vi "Handler - Set APU&ECU Cntrls.vi"(8 "error in (no error)":errorcluster, 10 "APU & ECU Controls":T1, 11 "Message Handler Loop Data in":T2) -> (0 "error out":errorcluster)   [LabVIEW 2018]
uses:
  Private Controls/Message Handler Loop Data.ctl
  Modules/Testing UI 1/Private Controls/APU & ECU Controls.ctl
  Modules/Testing UI 1/Testing UI 1.lvlib
  FPGA/FPGA VI Reference.ctl
panel:
  # "GTCP331-200ER Control Panel Discrete Input Panel"
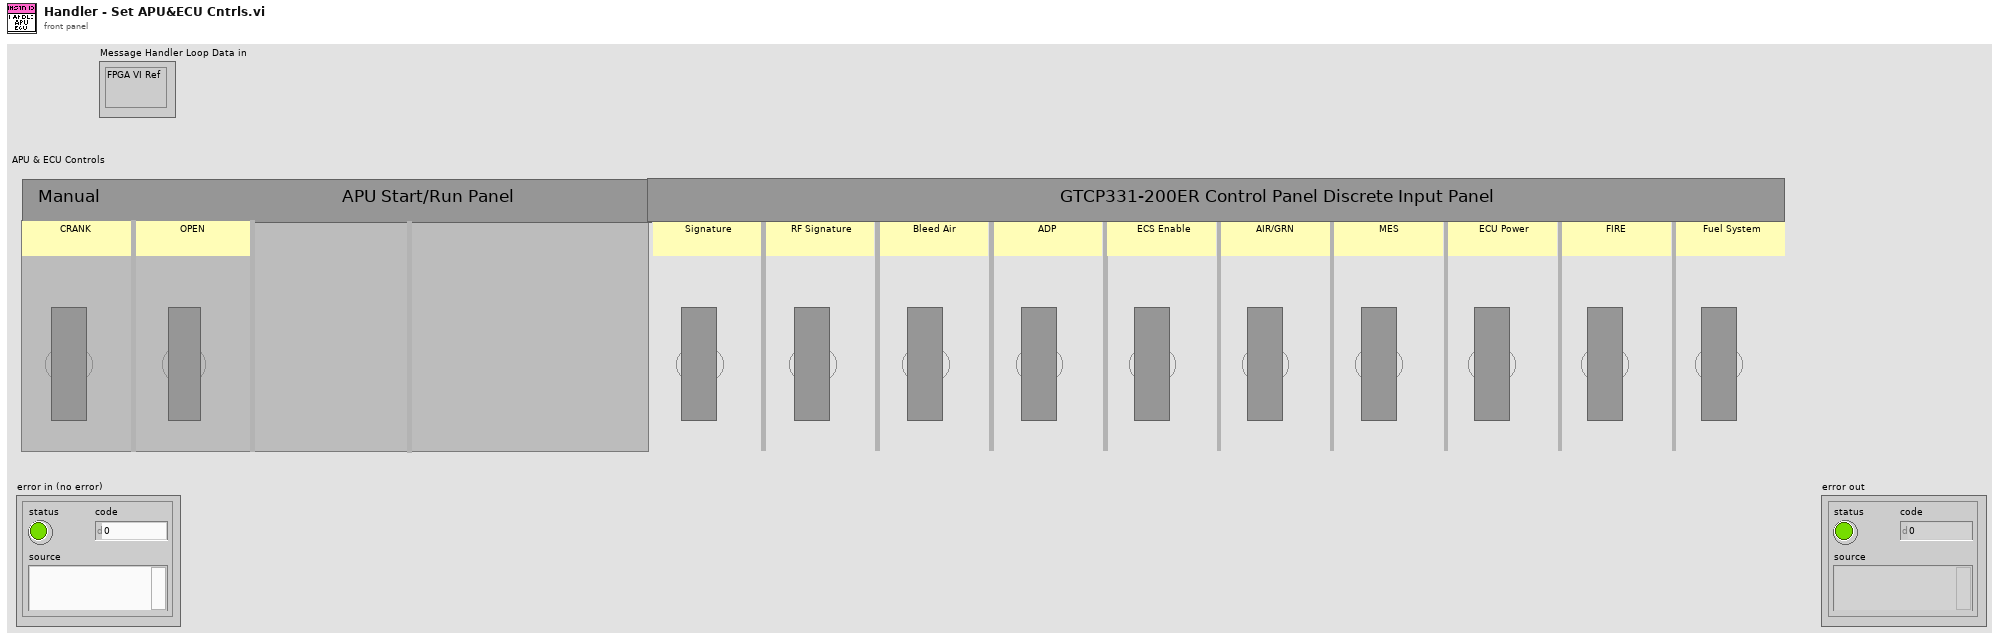
[diagram p1: front panel]
types:
  T1 = typedef "Testing UI 1.lvlib/APU & ECU Controls.ctl" = cluster{"02.00.9485.00":bool, "02.01.9485.03":bool, "02.01.9485.00":bool, "02.01.9485.01":bool, "02.00.9485.01":bool, "02.00.9485.02":bool, "02.00.9485.03":bool, "02.00.9485.04":bool, "02.00.9485.05":bool, "02.01.9485.06":bool, "02.00.9485.07":bool, "00.04.9265.03":bool}
  T2 = typedef "RT - Instrument IO.lvlib/Message Handler Loop Data.ctl" = cluster{"FPGA VI Ref":T3}
  T3 = typedef "FPGA VI Reference.ctl" = refnum<k20>
  T4 = cluster{"02.00.9485.00":bool, "02.01.9485.06":bool, "02.01.9485.00":bool, "02.01.9485.01":bool, "02.00.9485.01":bool, "02.00.9485.02":bool, "02.00.9485.03":bool, "02.00.9485.04":bool, "02.00.9485.05":bool, "02.00.9485.07":bool, "00.04.9265.03":sgl}
  T5 = typedef "Parsed Tag Cluster.ctl" = cluster{"Whole Tag":string, "# of Sections":u8, "Chassis":u8, "Slot":u8, "Module":string, "Channel":u8, "SubChannel":u8}
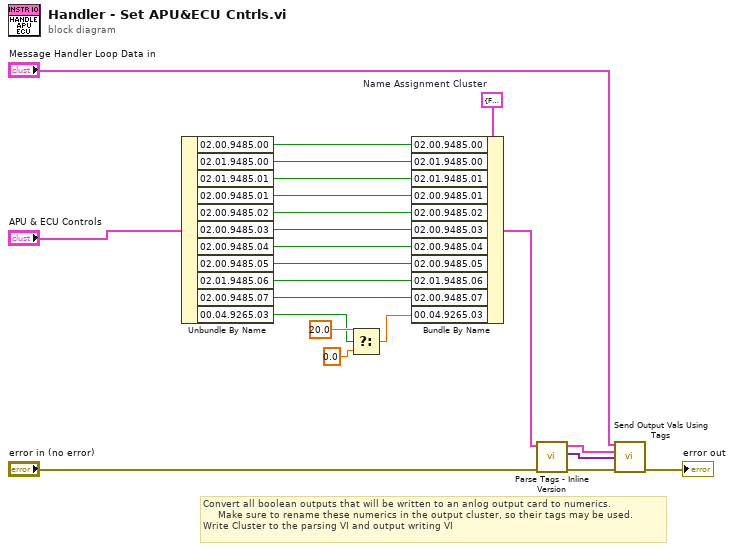
[diagram p0: block diagram]
diagram:
  w6 = T4 {"02.00.9485.00"=FALSE, "02.01.9485.06"=FALSE, "02.01.9485.00"=FALSE, "02.01.9485.01"=FALSE, "02.00.9485.01"=FALSE, "02.00.9485.02"=FALSE, "02.00.9485.03"=FALSE, "02.00.9485.04"=FALSE, "02.00.9485.05"=FALSE, "02.00.9485.07"=FALSE, "00.04.9265.03"=0.0}  # Name Assignment Cluster
  # "Convert all boolean outputs that will be written to an anlog output card to numerics.\n     Make sure to rename these numerics in the output cluster, so their tags may be used.\nWrite Cluster to the parsing VI and output writing VI"
  n1 = Unbundle By Name("APU & ECU Controls") -> ("02.00.9485.00"=w16:bool, "02.01.9485.00"=w15:bool, "02.01.9485.01"=w14:bool, "02.00.9485.01"=w13:bool, "02.00.9485.02"=w12:bool, "02.00.9485.03"=w11:bool, "02.00.9485.04"=w10:bool, "02.00.9485.05"=w9:bool, "02.01.9485.06"=w1:bool, "02.00.9485.07"=w8:bool, "00.04.9265.03"=w20:bool)
  n2 = Select(t=sgl 20.0 ("new element/subarray"), s=w20, f=sgl 0.0 ("new element/subarray")) -> (s? t:f=w7:sgl)
  n3 = Bundle By Name(cluster=w6, "02.00.9485.00"=w16, "02.01.9485.00"=w15, "02.01.9485.01"=w14, "02.00.9485.01"=w13, "02.00.9485.02"=w12, "02.00.9485.03"=w11, "02.00.9485.04"=w10, "02.00.9485.05"=w9, "02.01.9485.06"=w1, "02.00.9485.07"=w8, "00.04.9265.03"=w7) -> (w5:T4)
  n4 = call "Parse Tags - Inline Version.vi"("error in (no error)"="error in (no error)", "Cluster of Controls"=w5) -> ("error out"=w19:errorcluster, "[VData out]"=w17:variant[], "[Parsed Tags]"=w18:T5[])  [unwired: 6 in, 1 out]
  n5 = call "Send Output Vals Using Tags.vi"("Message Handler Loop Data in"="Message Handler Loop Data in", "[Parsed Tags]"=w18, "Array of VData in"=w17, "error in (no error)"=w19) -> ("error out"=→"error out":errorcluster)  [unwired: 11 in]
